vi "Modulo.vi"(1 "y":dbl, 2 "x":dbl) -> (0 "x%y":dbl)   [LabVIEW 2014]
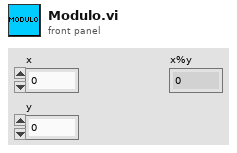
[diagram p1: front panel]
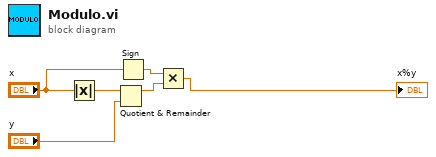
[diagram p0: block diagram]
diagram:
  n1 = Absolute Value(x="x") -> (abs(x)=w6:dbl)
  n2 = Quotient & Remainder(x=w6, y="y") -> (x-y*floor(x/y)=w2:dbl)  [unwired: 1 out]
  n3 = Sign(1:"x") -> (0:w3:dbl)
  n4 = Multiply(x=w3, y=w2) -> (x*y=→"x%y":dbl)
